vi "Find Expected Controls.vi"(8 "error in":errorcluster, 11 "vi info":T1 {"RegisterMap"."Address" format="%.0x"}) -> (0 "error out":errorcluster, 1 "Use?":bool, 2 "Controls":T8[](array[typedef]) {"Data Type" format="%.0x"}, 3 "Indicator":T8[](array[typedef]) {"Data Type" format="%.0x"}, 5 "Groups":string[](array[string]))   [LabVIEW 2015, in "Fuel Injector Analysis Addon System Explorer.lvlib"]
uses:
  Fuel Injector Analysis Addon System Explorer.lvlib
  Shared/Types/Register.Info.ctl
  Shared/Types/FPGA Data Types.ctl
  <vilib>/rvi/Bitfile/niFpgaBitfileStructure_VI.ctl
  <vilib>/rvi/Bitfile/nirviControlStructure.ctl
  <vilib>/rvi/Bitfile/nirviTypdefDescription.ctl
  <vilib>/rvi/Bitfile/nirviMechanicalAction.ctl
  <vilib>/rvi/Bitfile/nirviSubControlStructure.ctl
  <vilib>/rvi/Bitfile/nirviClusterElementControl.ctl
  <vilib>/picture/picture.llb/imagedata.ctl
  FPGA/Injection Capture IP/Types/Injection.Global.Settings.ctl
  FPGA/Injection Capture IP/Types/Injection.Timing.ctl
  FPGA/Injection Capture IP/Types/Injection.Core.Settings.ctl
  Shared/Fuel Injector Analysis Addon Shared.lvlib
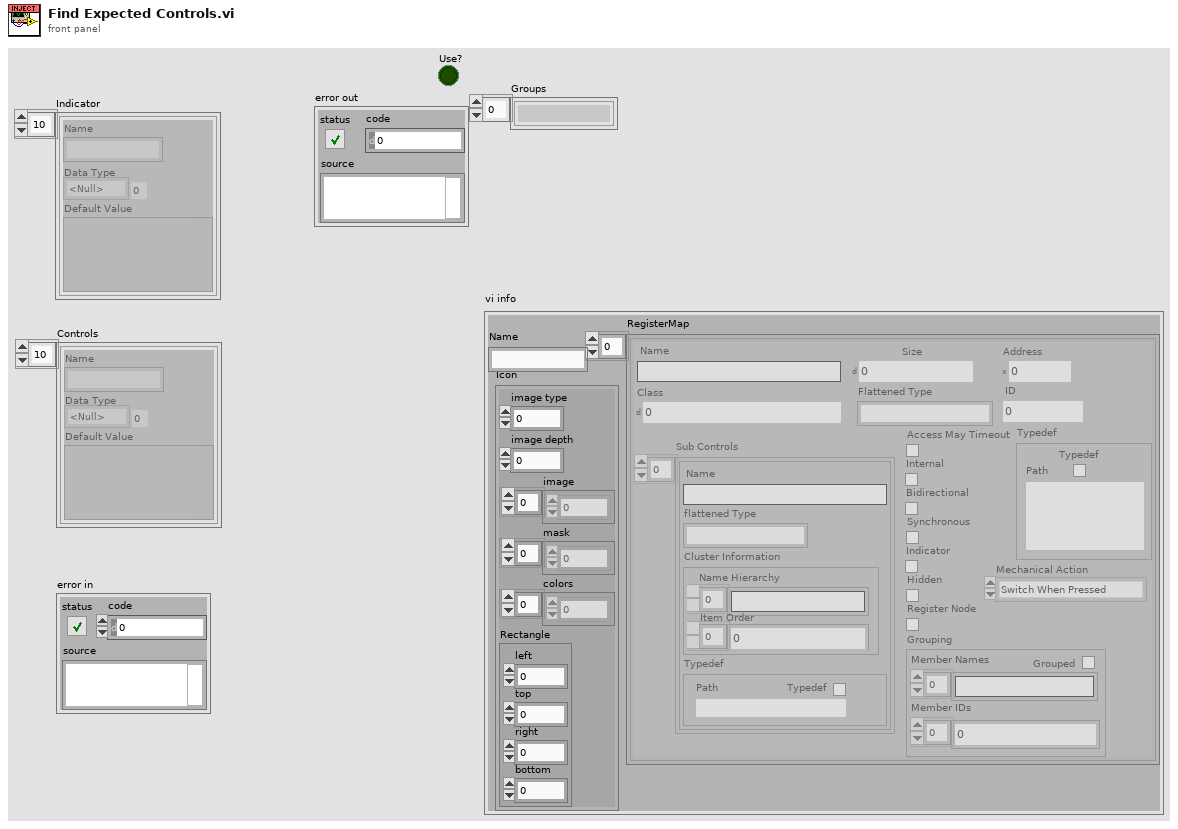
[diagram p1: front panel]
types:
  T1 = typedef "niFpgaBitfileStructure_VI.ctl" = cluster{"Name":string, "RegisterMap":T2[], "Icon":T7}
  T2 = typedef "nirviControlStructure.ctl" = cluster{"Name":string, "Hidden":bool, "Indicator":bool, "Flattened Type":string, "Grouping":cluster{"Grouped":bool, "Member Names":string[], "Member IDs":u32[]}, "Address":u32, "Size":u32, "Class":u32, "Internal":bool, "Typedef":T3, "ID":u32, "Bidirectional":bool, "Synchronous":bool, "Mechanical Action":T4, "Sub Controls":T5[], "Access May Timeout":bool, "Register Node":bool}
  T3 = typedef "nirviTypdefDescription.ctl" = cluster{"Typedef":bool, "Path":path}
  T4 = typedef "nirviMechanicalAction.ctl" = enum8{"Switch When Pressed", "Switch When Released", "Switch Until Released", "Latch When Pressed", "Latch When Released", "Latch Until Released"}
  T5 = typedef "nirviSubControlStructure.ctl" = cluster{"Name":string, "flattened Type":string, "Cluster Information":T6, "Typedef":T3}
  T6 = typedef "nirviClusterElementControl.ctl" = cluster{"Name Hierarchy":string[], "Item Order":u32[]}
  T7 = typedef "imagedata.ctl" = cluster{"image type":i32, "image depth":i32, "image":u8[], "mask":u8[], "colors":u32[], "Rectangle":cluster{"left":i16, "top":i16, "right":i16, "bottom":i16}}
  T8 = typedef "Fuel Injector Analysis Addon Shared.lvlib/Register.Info.ctl" = cluster{"Name":string, "Data Type":T9, "Default Value":variant}
  T9 = typedef "Fuel Injector Analysis Addon Shared.lvlib/FPGA Data Types.ctl" = enum8{"<Null>", "Injector.Core.Setting", "Injector.Global.Setting", "Injector.Mux.Setting", "Injector.Timing"}
  T10 = typedef "Injection.Core.Settings.ctl" = cluster{"Voltage Offset":fxp<+/-,32,8>, "Current Offset":fxp<+/-,32,8>}
  T11 = typedef "Injection.Timing.ctl" = cluster{"Injection Sample Period (Ticks)":u32}
  T12 = typedef "Injection.Global.Settings.ctl" = cluster{"Enable?":bool, "Initial Voltage Threshold":fxp<+/-,32,8>, "Event Dwell Limit":u16, "Voltage Gain":fxp<+/-,32,8>, "Current Gain":fxp<+/-,32,8>, "Filter Samples":u8, "Pretrigger Samples":u8}
  T13 = typedef "Type Descriptor Enumeration__ogtk.ctl" = enum8{"<Null>", "I8", "I16", "I32", "I64", "U8", "U16", "U32", "U64", "SGL", "DBL", "EXT", "CSG", "CDB", "CXT", "0x0F", "0x10", "0x11", "0x12", "0x13", "0x14", "Enum U8", "Enum U16", "Enum U32", "Enum U64", "SGL PQ", "DBL PQ", "EXT PQ", "CSG PQ", "CDB PQ", "CXT PQ", "0x1F", "0x20", "Boolean", "0x22", "0x23", "0x24", "0x25", "0x26", "0x27", "0x28", "0x29", "0x2A", "0x2B", "0x2C", "0x2D", "0x2E", "0x2F", "String", "0x31", "Path", "Pict", "0x34", "0x35", "0x36", "DAQ", "0x38", "0x39", "0x3A", "0x3B", "0x3C", "0x3D", "0x3E", "0x3F", "Array", "0x41", "0x42", "0x43", "0x44", "0x45", "0x46", "0x47", "0x48", "0x49", "0x4A", "0x4B", "0x4C", "0x4D", "0x4E", "0x4F", "Cluster", "0x51", "0x52", "Variant", "Waveform", "0x55", "0x56", "0x57", "0x58", "0x59", "0x5A", "0x5B", "0x5C", "0x5D", "0x5E", "0x5F", "0x60", "0x61", "0x62", "0x63", "0x64", "0x65", "0x66", "0x67", "0x68", "0x69", "0x6A", "0x6B", "0x6C", "0x6D", "0x6E", "0x6F", "Refnum"}
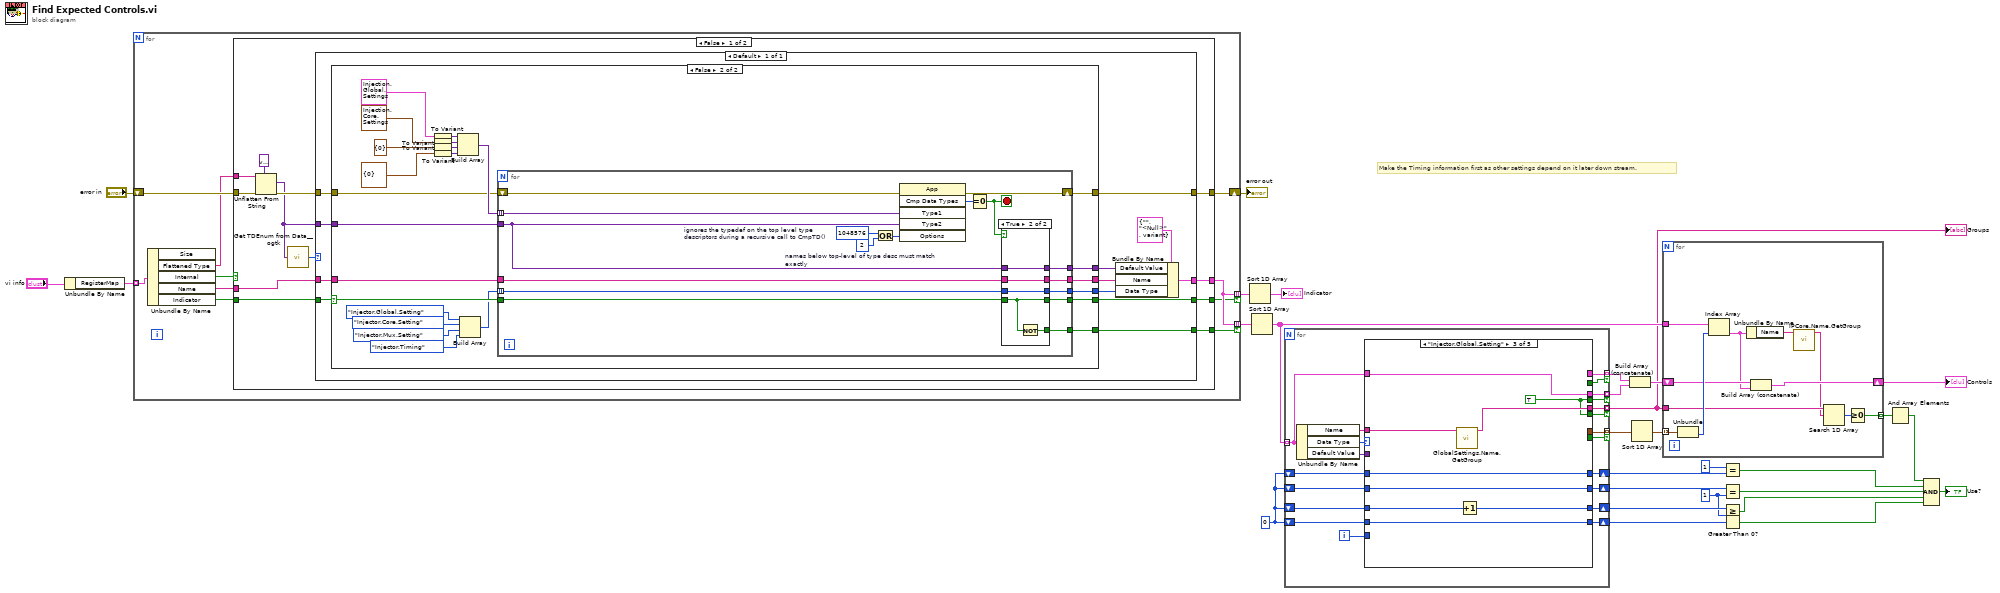
[diagram p0: block diagram]
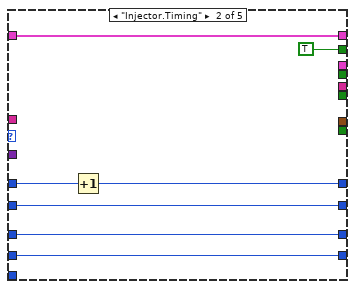
[diagram p3: hidden frame]
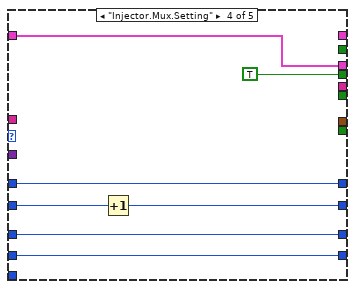
[diagram p4: hidden frame]
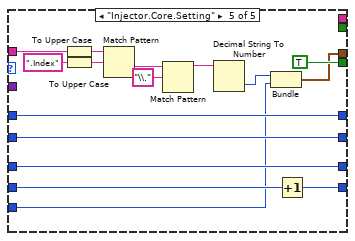
[diagram p5: hidden frame]
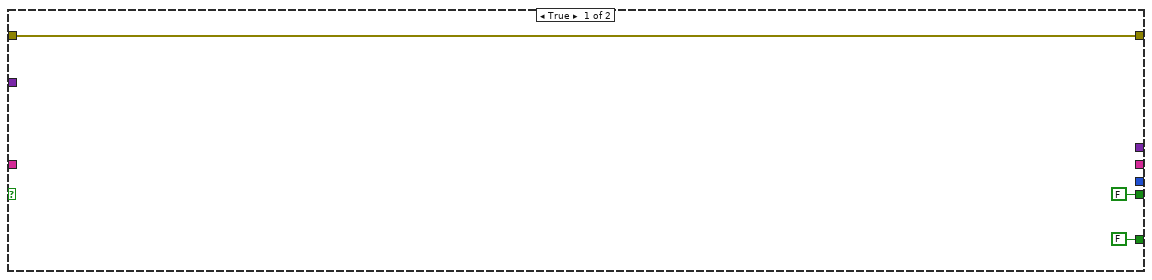
[diagram p6: hidden frame]
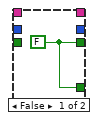
[diagram p7: hidden frame]
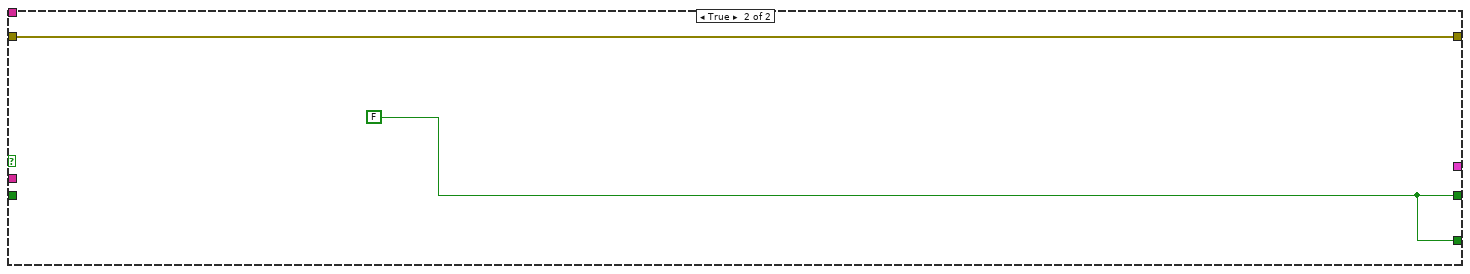
[diagram p8: hidden frame]
diagram:
  w14 = 1 ("y")
  w17 = 0
  # "Make the Timing information first as other settings depend on it later down stream."
  n1 = Unbundle By Name("vi info") -> ("RegisterMap"=w28:T2[])
  n2 = for {
    tunnel: w28 -> [w34] mode=indexing
    tunnel: [w39] -> w29 mode=indexing if=w38
    tunnel: [w39] -> w11 mode=indexing if=w37
    shift-right: [w36] -> w25
    shift-left: "error in" -> [w35]
    n3 = Unbundle By Name(w34) -> ("Flattened Type"=w30:string, "Internal"=w31:bool, "Name"=w32:string, "Indicator"=w33:bool)  [unwired: 1 out]
    n4 = case shown="False" w31 {
      tunnel: w32 -> [w50 _]
      tunnel: w33 -> [w49 _]
      tunnel: [w48 _] -> w39
      tunnel: [w47 w115] -> w38
      tunnel: [w46 w115] -> w37
      tunnel: w30 -> [w43 _]
      tunnel: [w45 w114] -> w36
      tunnel: w35 -> [w42 w114]
      frame False {
        n5 = Unflatten From String(type=variant ("Variant"), binary string=w43, error in (no error)=w42) -> (value=w40:variant, error out=w41:errorcluster)  [unwired: 3 out]
        n6 = call <userlib>:"Get TDEnum from Data__ogtk.vi"("Data"=w40) -> ("Type Descriptor Enumeration"=w51:T13)  [unwired: 4 in]
        n7 = case shown="Default" w51 {
          tunnel: [w63] -> w47
          tunnel: w49 -> [w58]
          tunnel: w50 -> [w59]
          tunnel: [w60] -> w48
          tunnel: [w62] -> w46
          tunnel: w40 -> [w57]
          tunnel: [w53] -> w45
          tunnel: w41 -> [w52]
          frame Default {
            n8 = case shown="False" w58 {
              selector: w58 -> [_ w87]
              tunnel: [FALSE ("Boolean") w90] -> w63
              tunnel: [FALSE ("Boolean") w89] -> w62
              tunnel: w59 -> [_ w88]
              tunnel: w57 -> [_ w83]
              tunnel: [_ w82] -> w56
              tunnel: [_ w81] -> w55
              tunnel: [_ w80] -> w54
              tunnel: [w66 w75] -> w53
              tunnel: w52 -> [w66 w76]
              frame True {
              }
              frame False {
                n9 = To Variant(anything=T12 {"Enable?"=FALSE, "Initial Voltage Threshold"=0.0, "Event Dwell Limit"=0, "Voltage Gain"=0.0, "Current Gain"=1.0, "Filter Samples"=5, "Pretrigger Samples"=5} ("InjectorAnalysis.Settings")) -> (Variant=w86:variant)
                n10 = To Variant(anything=T10 {"Voltage Offset"=0.0, "Current Offset"=0.0} ("Index<#>.<UserName>")) -> (Variant=w78:variant)
                n11 = To Variant(anything=cluster{"# of Injectors":u8} {"# of Injectors"=0} ("Injector.MUX.Settings")) -> (Variant=w77:variant)
                n12 = To Variant(anything=T11 {"Injection Sample Period (Ticks)"=0} ("Injector.Timing")) -> (Variant=w74:variant)
                n13 = Build Array(w86, w78, w77, w74) -> (w84:variant[])
                n14 = Build Array(FPGA_Data_Types."Injector.Global.Setting" ("Data Type"), FPGA_Data_Types."Injector.Core.Setting" ("Data Type"), FPGA_Data_Types."Injector.Mux.Setting" ("Data Type"), FPGA_Data_Types."Injector.Timing" ("Data Type")) -> (w79:T9[])
                n15 = for {
                  tunnel: w83 -> [w96]
                  tunnel: [w105] -> w89
                  tunnel: w88 -> [w104]
                  tunnel: w84 -> [w95] mode=indexing
                  tunnel: [w103] -> w81
                  tunnel: [w102] -> w82
                  tunnel: [w101] -> w80
                  tunnel: w79 -> [w100] mode=indexing
                  tunnel: w87 -> [w107]
                  tunnel: [w106] -> w90
                  shift-right: [w91] -> w75
                  shift-left: w76 -> [w92]
                  stop <- w93 stop-if-true
                  w98 = 2  # names below top-level of type desc must match exactly
                  w97 = 1048576  # ignores the typedef on the top level type descriptors during a recursive call to CmpTD()
                  n16 = Or(x=w97, y=w98) -> (x .or. y?=w99:i32)
                  n17 = invoke class="App" method="Cmp Data Types"(error in=w92, "Type1"=w95, "Type2"=w96, "Options"=w99) -> (error out=w91:errorcluster, "Compare Data Types"=w94:i32)  [unwired: 2 in, 4 out]
                  n18 = Equal To 0?(x=w94) -> (x = 0?=w93:bool)
                  n19 = case shown="True" w93 {
                    tunnel: w107 -> [_ w113]
                    tunnel: [w108 w113] -> w106
                    tunnel: [w108 w112] -> w105
                    tunnel: w104 -> [_ w110]
                    tunnel: [_ w111] -> w103
                    tunnel: w96 -> [_ w111]
                    tunnel: [_ w110] -> w102
                    tunnel: [_ w109] -> w101
                    tunnel: w100 -> [_ w109]
                    frame False {
                      w108 = FALSE ("Boolean")
                    }
                    frame True {
                      n20 = Not(x=w113) -> (.not. x?=w112:bool)
                    }
                  }
                }
              }
            }
            n21 = Bundle By Name(cluster=T8 {"Name"="", "Data Type"=enum."<Null>", "Default Value"=variant(refnum<class> refnum)}, "Default Value"=w55, "Name"=w56, "Data Type"=w54) -> (w60:T8)
          }
        }
      }
      frame True {
        w115 = FALSE ("Boolean")
      }
    }
  }
  "error out" <- w25
  n22 = Sort 1D Array(array=w29) -> (sorted array=→"Indicator":T8[])
  n23 = Sort 1D Array(array=w11) -> (sorted array=w9:T8[])
  n24 = for {
    tunnel: w9 -> [w122] mode=indexing
    shift-right: [w134] -> w16
    shift-left: w17 -> [w135]
    shift-right: [w133] -> w21
    shift-left: w17 -> [w132]
    shift-right: [w130] -> w15
    shift-left: w17 -> [w129]
    shift-right: [w127] -> w23
    shift-left: w17 -> [w128]
    tunnel: [w125] -> w10 mode=indexing if=w124
    tunnel: [w121] -> w6 mode=indexing if=w120
    tunnel: [w119] -> w5 mode=indexing if=w117
    tunnel: [w118] -> w3 mode=indexing if=w116
    i -> [w123]
    n25 = Unbundle By Name(w122) -> ("Name"=w126:string, "Data Type"=w136:T9, "Default Value"=w131:variant)
    n26 = case shown="\"Injector.Global.Setting\"" w136 {
      tunnel: w135 -> [w140 w147 w156 w163 w179]
      tunnel: [w140 w147 w156 w163 w178] -> w134
      tunnel: [w139 w146 w154 w162 w177] -> w133
      tunnel: w132 -> [w139 w146 w155 w162 w177]
      tunnel: w131 -> [_ _ _ _ _]
      tunnel: [w138 w145 w153 w159 w176] -> w130
      tunnel: w129 -> [w138 w145 w153 w160 w176]
      tunnel: w128 -> [w137 w144 w152 w161 w175]
      tunnel: [w137 w143 w152 w161 w175] -> w127
      tunnel: [_ _ _ _ TRUE] -> w124
      tunnel: w126 -> [_ _ w150 _ w173]
      tunnel: [_ _ _ _ w165] -> w125
      tunnel: w123 -> [_ _ _ _ w164]
      tunnel: w122 -> [_ w142 w151 w158 _]
      tunnel: [_ w142 _ _ _] -> w121
      tunnel: [_ TRUE _ _ _] -> w120
      tunnel: [_ _ w151 w158 _] -> w119
      tunnel: [_ _ w148 TRUE _] -> w117
      tunnel: [_ _ w149 _ _] -> w118
      tunnel: [_ _ w148 _ _] -> w116
      frame "<Null>", Default {
      }
      frame "Injector.Timing" {
        n27 = Increment(x=w144) -> (x+1=w143:i32)
      }
      frame "Injector.Global.Setting" {
        w148 = TRUE
        n28 = call "GlobalSettings.Name.GetGroup.vi"("Name"=w150) -> ("Group"=w149:string)  [unwired: 10 in]
        n29 = Increment(x=w155) -> (x+1=w154:i32)
      }
      frame "Injector.Mux.Setting" {
        n30 = Increment(x=w160) -> (x+1=w159:i32)
      }
      frame "Injector.Core.Setting" {
        n31 = To Upper Case(1:w173) -> (0:w171:string)
        n32 = To Upper Case(1:".Index" ("regular expression")) -> (0:w170:string)
        n33 = Match Pattern(string=w171, regular expression=w170) -> (after substring=w169:string)  [unwired: 1 in, 3 out]
        n34 = Match Pattern(string=w169, regular expression="\\.") -> (before substring=w167:string)  [unwired: 1 in, 3 out]
        n35 = Decimal String To Number(string=w167) -> (number=w166:i32)  [unwired: 2 in, 1 out]
        n36 = Bundle(w166, w164) -> (w165:cluster{i32, i32})  [unwired: 1 in]
        n37 = Increment(x=w179) -> (x+1=w178:i32)
      }
    }
  }
  "Groups" <- w3
  n38 = Build Array (concatenate)(w6, w5) -> (w4:T8[])
  n39 = Sort 1D Array(array=w10) -> (sorted array=w8:cluster{i32, i32}[])
  n40 = for {
    shift-right: [w186] -> w7
    shift-left: w4 -> [w187]
    tunnel: w9 -> [w190]
    tunnel: w8 -> [w189] mode=indexing
    tunnel: w3 -> [w183]
    tunnel: [w180] -> w2 mode=indexing
    n41 = Unbundle(w189) -> (w188:i32)  [unwired: 1 out]
    n42 = Index Array(array=w190, index=w188) -> (element=w185:T8)
    n43 = Unbundle By Name(w185) -> ("Name"=w184:string)
    n44 = Build Array (concatenate)(w187, w185) -> (w186:T8[])
    n45 = call "IPCore.Name.GetGroup.vi"("Name"=w184) -> ("Group"=w182:string)  [unwired: 10 in]
    n46 = Search 1D Array(1D array=w183, element=w182) -> (index of element=w181:i32)  [unwired: 1 in]
    n47 = Greater Or Equal To 0?(x=w181) -> (x >= 0?=w180:bool)
  }
  "Controls" <- w7
  n48 = Equal?(x=1 ("y"), y=w23) -> (x = y?=w19:bool)
  n49 = Equal?(x=w15, y=w14) -> (x = y?=w12:bool)
  n50 = Greater Or Equal?(x=w21, y=w14) -> (x >= y?=w13:bool)
  n51 = Greater Than 0?(x=w16) -> (x > 0?=w20:bool)
  n52 = And Array Elements(Boolean array=w2) -> (logical AND=w1:bool)
  n53 = Compound Arithmetic op=AND(w1, w19, w12, w13, w20) -> (→"Use?":bool)
